vi "USB9825_AD_Link.vi"(8 "Error In":errorcluster caption="错误输入") -> (0 "Error Out":errorcluster caption="错误输出", 1 "DevNum":i32, 2 "设备属性":string, 3 "hDevice":i32)   [LabVIEW 2015, in "DAQ.lvlib"]
uses:
  DAQ.lvlib
  USB9825.DLL
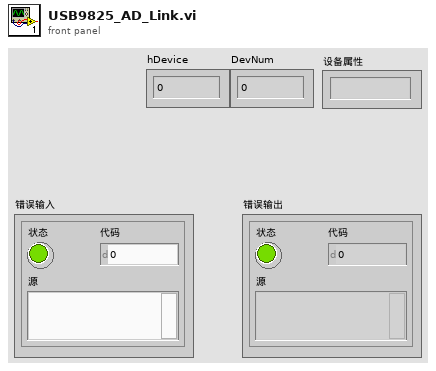
[diagram p1: front panel]
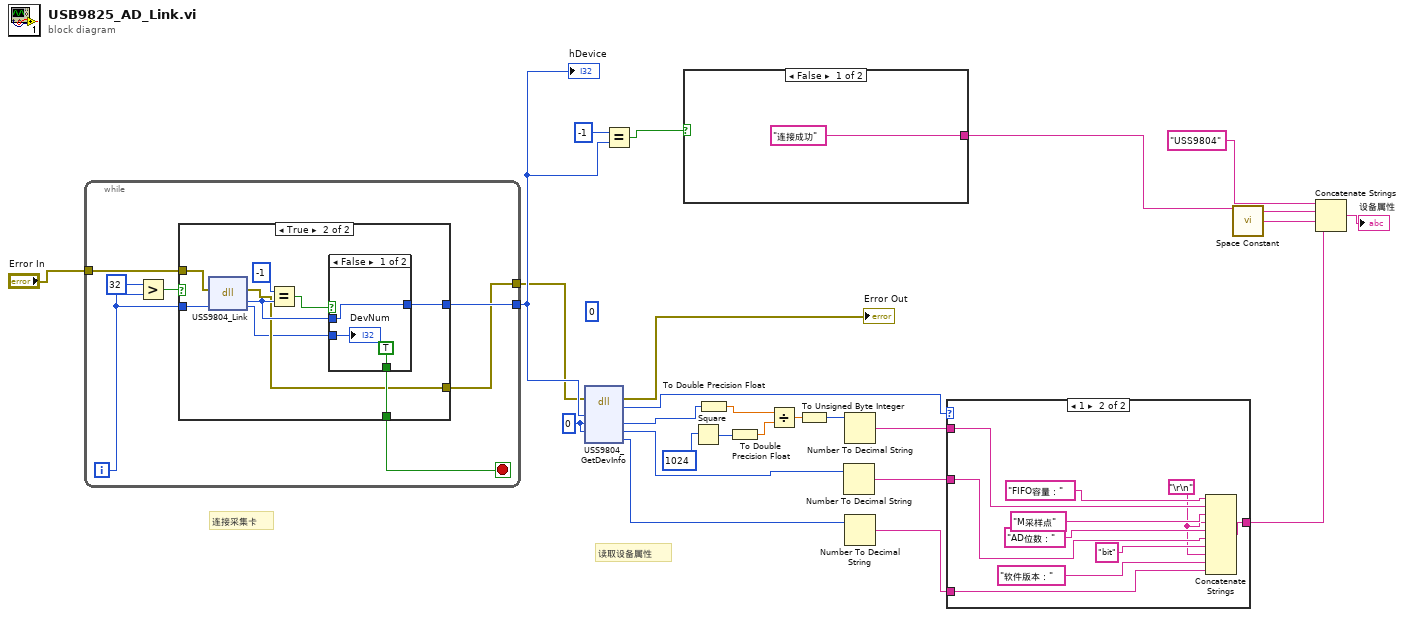
[diagram p0: block diagram]
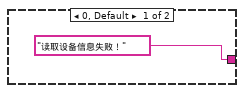
[diagram p2: hidden frame]
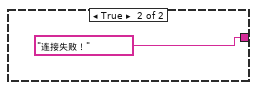
[diagram p3: hidden frame]
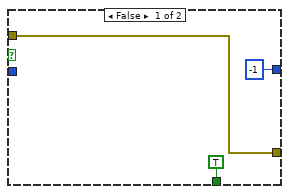
[diagram p4: hidden frame]
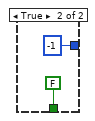
[diagram p5: hidden frame]
diagram:
  w25 = 0 ("devFifoSize")
  (unwired) u8 0 ("pDat")
  # "读取设备属性"
  # "连接采集卡"
  n1 = while {
    tunnel: [w29] -> w24
    tunnel: "Error In" -> [w27]
    tunnel: [w26] -> w3
    i -> [w30]
    stop <- w28 stop-if-true
    n2 = Greater?(x=32, y=w30) -> (0:w32:bool)
    n3 = case shown="True" w32 {
      tunnel: w30 -> [_ w44]
      tunnel: [-1 ("返回类型") w41] -> w29
      tunnel: [TRUE w39] -> w28
      tunnel: w27 -> [w33 w38]
      tunnel: [w33 w37] -> w26
      frame False {
      }
      frame True {
        n4 = dll-call lib="PTH2sabs CYexinrongWorkplace\t普密斯Thickness-measurementBiometry_alpha3 bolihouduSub VIsDAQUSB9825.dll" fn="USS9804_Link"(error in=w38, "DevNum"=w44) -> (error out=w37:errorcluster, "返回类型"=w40:i32, "DevNum"=w36:u8)  [unwired: 2 in, 1 out]
        n5 = Equal?(x=-1, y=w40) -> (x = y?=w42:bool)
        n6 = case shown="False" w42 {
          tunnel: [w47 -1 ("返回类型")] -> w41
          tunnel: w40 -> [w47 _]
          tunnel: [TRUE FALSE] -> w39
          tunnel: w36 -> [w45 _]
          frame False {
            "DevNum" <- w45
          }
          frame True {
          }
        }
      }
    }
  }
  "hDevice" <- w24
  n7 = dll-call lib="PTH2sabs CYexinrongWorkplace\t普密斯Thickness-measurementBiometry_alpha3 bolihouduSub VIsDAQUSB9825.dll" fn="USS9804_GetDevInfo"(error in=w3, "hDevice"=w24, "devFifoSize"=w25, "devADbit"=w25) -> (error out=→"Error Out":errorcluster, "返回类型"=w22:i32, "devFifoSize"=w20:i32, "devADbit"=w13:i32, "devVer"=w2:i32)  [unwired: 4 in, 1 out]
  n8 = Equal?(x=-1, y=w24) -> (x = y?=w4:bool)
  n9 = case shown="False" w4 {
    tunnel: ["连接成功" "连接失败！"] -> w10
    frame False {
    }
    frame True {
    }
  }
  n10 = Square(x=u32 1024) -> (x^2=w17:u32)
  n11 = To Double Precision Float(number=w20) -> (double precision float=w19:dbl)
  n12 = To Double Precision Float(number=w17) -> (double precision float=w16:dbl)
  n13 = Divide(x=w19, y=w16) -> (x/y=w18:dbl)
  n14 = To Unsigned Byte Integer(number=w18) -> (unsigned 8bit integer=w15:u8)
  n15 = Number To Decimal String(number=w13) -> (decimal integer string=w12:string)  [unwired: 1 in]
  n16 = Number To Decimal String(number=w15) -> (decimal integer string=w14:string)  [unwired: 1 in]
  n17 = Number To Decimal String(number=w2) -> (decimal integer string=w1:string)  [unwired: 1 in]
  n18 = case shown="1" w22 {
    tunnel: w14 -> [_ w58]
    tunnel: w12 -> [_ w57]
    tunnel: ["读取设备信息失败！" w56] -> w8
    tunnel: w1 -> [_ w53]
    frame 0, Default {
    }
    frame 1 {
      w55 = "\r\n"
      n19 = Concatenate Strings("FIFO容量：", w58, "M采样点", w55, "AD位数：", w57, "bit", w55, "软件版本：" ("string"), w53) -> (w56:string)
    }
  }
  n20 = call <vilib>:"Space Constant.vi"() -> ("String"=w9:string)
  n21 = Concatenate Strings("USS9804", w10, w9, w8) -> (→"设备属性":string)
